vi "OldIntakeNetworkSlow.vi"(8 "error in (no error)":errorcluster) -> (0 "error out":errorcluster)   [LabVIEW 2023]
uses:
  OldIntakeGlobal.vi
  <vilib>/Rock Robotics/Network Tables/NT Read Number.vi
  <vilib>/Rock Robotics/Network Tables/NT Write Number.vi
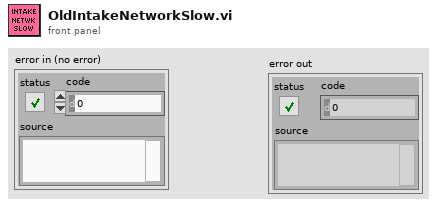
[diagram p1: front panel]
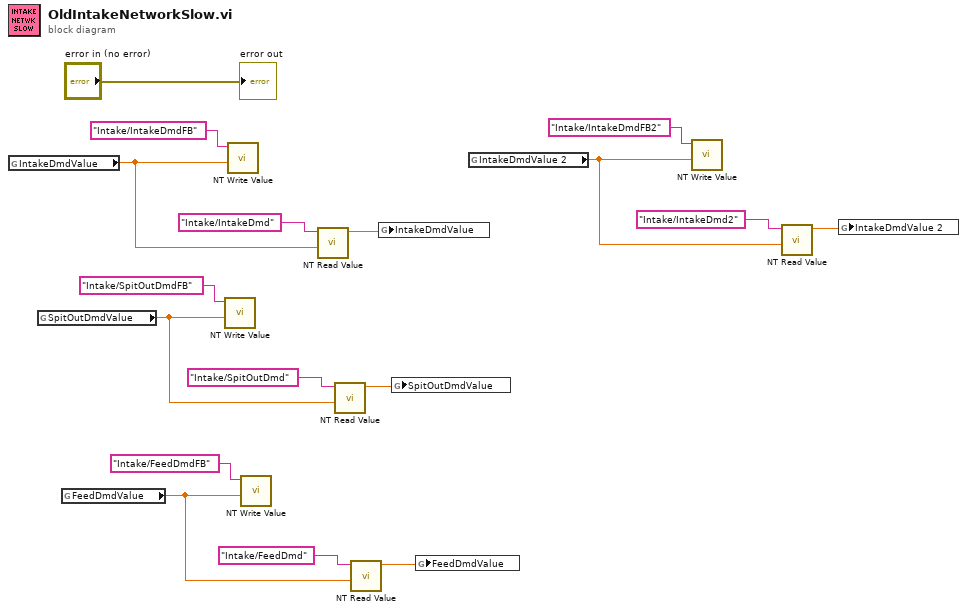
[diagram p0: block diagram]
diagram:
  n1 = global read "OldIntakeGlobal.vi" "IntakeDmdValue"() -> (w12:dbl)
  n2 = global read "OldIntakeGlobal.vi" "SpitOutDmdValue"() -> (w9:dbl)
  n3 = global read "OldIntakeGlobal.vi" "FeedDmdValue"() -> (w5:dbl)
  n4 = call-poly <vilib>:"NT Write Value.vi"("value"=w9, "name"="Intake/SpitOutDmdFB") -> ()  [unwired: 9 in, 1 out]
  n5 = call-poly <vilib>:"NT Write Value.vi"("value"=w12, "name"="Intake/IntakeDmdFB") -> ()  [unwired: 9 in, 1 out]
  n6 = call-poly <vilib>:"NT Write Value.vi"("value"=w5, "name"="Intake/FeedDmdFB") -> ()  [unwired: 9 in, 1 out]
  n7 = call-poly <vilib>:"NT Read Value.vi"("default value"=w12, "name"="Intake/IntakeDmd") -> ("value"=w13:dbl)  [unwired: 7 in, 2 out]
  n8 = call-poly <vilib>:"NT Read Value.vi"("default value"=w9, "name"="Intake/SpitOutDmd") -> ("value"=w10:dbl)  [unwired: 7 in, 2 out]
  n9 = call-poly <vilib>:"NT Read Value.vi"("default value"=w5, "name"="Intake/FeedDmd") -> ("value"=w6:dbl)  [unwired: 7 in, 2 out]
  n10 = global write "OldIntakeGlobal.vi" "IntakeDmdValue"(w13) -> ()
  n11 = global write "OldIntakeGlobal.vi" "SpitOutDmdValue"(w10) -> ()
  n12 = global write "OldIntakeGlobal.vi" "FeedDmdValue"(w6) -> ()
  n13 = global read "OldIntakeGlobal.vi" "IntakeDmdValue 2"() -> (w1:dbl)
  n14 = call-poly <vilib>:"NT Write Value.vi"("value"=w1, "name"="Intake/IntakeDmdFB2") -> ()  [unwired: 9 in, 1 out]
  n15 = call-poly <vilib>:"NT Read Value.vi"("default value"=w1, "name"="Intake/IntakeDmd2") -> ("value"=w2:dbl)  [unwired: 7 in, 2 out]
  n16 = global write "OldIntakeGlobal.vi" "IntakeDmdValue 2"(w2) -> ()
  "error out" <- "error in (no error)"
